vi "AMModEntry.vi"(0 "AMFreqSet":bool, 1 "Keypad In":dbl, 5 "AMFreq ini":dbl=1000.0, 7 "NumCycSet":bool, 9 "NumCyc ini":u16=1000, 11 "PkPwrSet":bool, 12 "PkPwr ini":dbl, 13 "AmpSet":bool, 14 "Amp ini":dbl=31.5) -> (3 "reset":bool, 4 "AM Freq":dbl=1000.0, 6 "NumCyc":u16=1000, 8 "PkPwr":dbl, 10 "Amplitude":dbl=31.5)   [LabVIEW 2017]
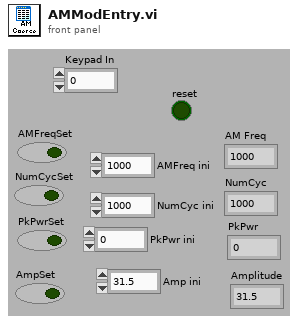
[diagram p1: front panel]
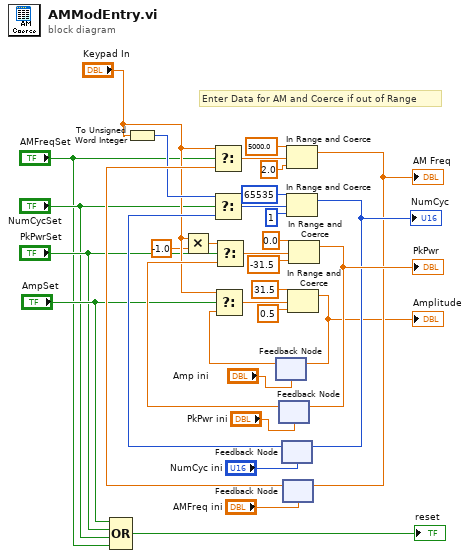
[diagram p0: block diagram]
diagram:
  # "Enter Data for AM and Coerce if out of Range"
  n1 = Compound Arithmetic op=OR("AmpSet", "PkPwrSet", "NumCycSet", "AMFreqSet") -> (→"reset":bool)
  n2 = To Unsigned Word Integer(number="Keypad In") -> (unsigned 16bit integer=w15:u16)
  n3 = Multiply(x="Keypad In", y=-1.0) -> (x*y=w8:dbl)
  n4 = feedback #1("Amp ini") -> (w10:dbl)
  n5 = Select(t="Keypad In", s="AmpSet", f=w10) -> (s? t:f=w13:dbl)
  n6 = feedback #2("PkPwr ini") -> (w26:dbl)
  n7 = Select(t=w8, s="PkPwrSet", f=w26) -> (s? t:f=w29:dbl)
  n8 = feedback #3("NumCyc ini") -> (w23:u16)
  n9 = Select(t=w15, s="NumCycSet", f=w23) -> (s? t:f=w31:u16)
  n10 = feedback #4("AMFreq ini") -> (w18:dbl)
  n11 = Select(t="Keypad In", s="AMFreqSet", f=w18) -> (s? t:f=w20:dbl)
  n12 = In Range and Coerce(upper limit=5000.0, x=w20, lower limit=2.0) -> (coerced(x)=w19:dbl)  [unwired: 1 out]
  "AM Freq" <- w19
  n13 = feedback-in #4(w19) -> ()
  n14 = In Range and Coerce(upper limit=u16 65535, x=w31, lower limit=u16 1) -> (coerced(x)=w24:u16)  [unwired: 1 out]
  "NumCyc" <- w24
  n15 = feedback-in #3(w24) -> ()
  n16 = In Range and Coerce(upper limit=31.5, x=w13, lower limit=0.5) -> (coerced(x)=w9:dbl)  [unwired: 1 out]
  "Amplitude" <- w9
  n17 = feedback-in #1(w9) -> ()
  n18 = In Range and Coerce(upper limit=0.0, x=w29, lower limit=-31.5) -> (coerced(x)=w27:dbl)  [unwired: 1 out]
  "PkPwr" <- w27
  n19 = feedback-in #2(w27) -> ()
